vi "Set Shutter TTL.vi"(8 "error in (no error)":errorcluster, 11 "CCDCamera in":refnum<class "CCDCamera.lvclass">) -> (0 "error out":errorcluster, 3 "CCDCamera out":refnum<class "CCDCamera.lvclass">)   [LabVIEW 2018, in "CCDCamera.lvclass"]
uses:
  CCDCamera.lvclass
  C:/Users/observer/Desktop/SPARC4_ACS/SPARC4_ACS/Simulated_CCD_Camera/Simulated_CCD_Camera.lvclass
  Simulated_CCD_Camera/Simulated_CCD_Camera.lvclass/Simulated_CCD_Camera.ctl
  Interface/Interface.lvclass
  Simulated_CCD_Camera/Simulated_CCD_Camera.lvclass
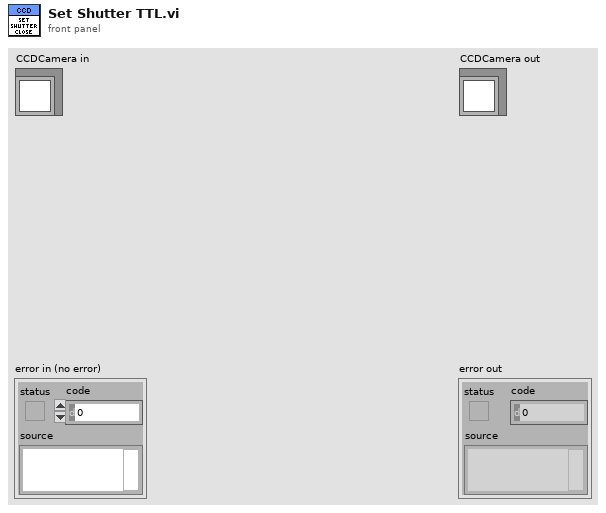
[diagram p1: front panel]
types:
  T1 = typedef "Shutter_mode typedef.ctl" = enum16{"Auto", "Open", "Close", "N/A (3)", "Open FVB Series", "Open Any Series"}
  T2 = typedef "ReadMode_mode typedef.ctl" = enum16{"Full Vertical Binning", "Multi-Track", "Random-Track", "Single-Track", "Image"}
  T3 = typedef "AcquisitionMode_mode typedef.ctl" = enum16{"Reserved (0)", "Single Scan", "Accumulate", "Kinetics", "Fast Kinetics", "Run Till Abort", "Reserved (6)", "Reserved (7)", "Reserved (8)", "Time Delayed Integration"}
  T4 = cluster{"PREAMP":enum16{"Gain 1", "Gain 2"}, "READOUT_RATE":enum16{"30 MHz", "20 MHz", "10 MHz", "1 MHz"}, "EM_GAIN":u16, "VBIN":u16, "INITIAL_LINE":u16, "INITIAL_COLUMN":u16, "FINAL_LINE":u16, "FINAL_COLUMN":u16, "TRIGGER_MODE":enum16{"Internal", "External", "N/A", "N/A_1", "N/A_2", "N/A_3", "External Start"}, "HBIN":u16, "SHUTTER_TTL":enum16{"TTL Low", "TTL High"}, "SHUTTER_MODE":T1, "SHUTTER_OPENING_TIME":u16, "SHUTTER_CLOSING_TIME":u16, "VERTICAL_SHIFT_SPEED":u16, "READ_MODE":T2, "FRAME_TRANSFER":bool, "VERTICAL_CLOCK_VOLTAGE":enum16{"0", "+1", "+2", "+3", "+4"}, "ACQUISITION_MODE":T3, "AD_CHANNEL":u16, "EM_MODE":enum16{"Electron Multiplying", "Conventional"}}
  T5 = cluster{"PREAMP":u16, "READOUT_RATE":u16, "EM_GAIN":u16, "VBIN":u16, "INITIAL_LINE":u16, "INITIAL_COLUMN":u16, "FINAL_LINE":u16, "FINAL_COLUMN":u16, "TRIGGER_MODE":u16, "HBIN":u16, "SHUTTER_TTL":u16, "SHUTTER_MODE":u16, "SHUTTER_OPENING_TIME":u16, "SHUTTER_CLOSING_TIME":u16, "VERTICAL_SHIFT_SPEED":u16, "READ_MODE":u16, "FRAME_TRANSFER":bool, "VERTICAL_CLOCK_VOLTAGE":u16, "ACQUISITION_MODE":u16, "AD_CHANNEL":u16, "EM_MODE":u16}
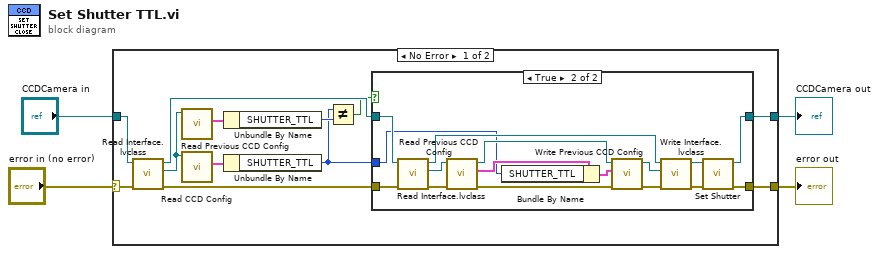
[diagram p0: block diagram]
diagram:
  n1 = case shown="No Error" "error in (no error)" {
    selector: "error in (no error)" -> [w16 w36]
    tunnel: [w13 w36] -> w1
    tunnel: [w12 w35] -> w2
    tunnel: "CCDCamera in" -> [w15 w35]
    frame No Error {
      n2 = call "Read Interface.lvclass.vi"("error in (no error)"=w16, "Simulated_CCD_Camera in"=w15) -> ("error out"=w11:errorcluster, "Interface.lvclass"=w5:refnum<class "Interface.lvclass">, "Simulated_CCD_Camera out"=w14:refnum<class "CCDCamera.lvclass">)  [unwired: 7 in]
      n3 = call "Read Previous CCD Config.vi"("Interface in"=w5) -> ("Previous CCD Config"=w9:T4)  [unwired: 8 in, 2 out]
      n4 = call "Read CCD Config.vi"("Interface in"=w5) -> ("Previous CCD Config"=w10:T5)  [unwired: 8 in, 2 out]
      n5 = Unbundle By Name(w9) -> ("SHUTTER_TTL"=w8:enum16{"TTL Low", "TTL High"})
      n6 = Unbundle By Name(w10) -> ("SHUTTER_TTL"=w6:u16)
      n7 = Not Equal?(x=w6, y=w8) -> (x != y?=w7:bool)
      n8 = case shown="True" w7 {
        tunnel: w14 -> [w18 w21]
        tunnel: [w17 w23] -> w13
        tunnel: [w18 w22] -> w12
        tunnel: w11 -> [w17 w20]
        tunnel: w6 -> [_ w19]
        frame False {
        }
        frame True {
          n9 = call "Read Interface.lvclass.vi"("error in (no error)"=w20, "Simulated_CCD_Camera in"=w21) -> ("error out"=w26:errorcluster, "Interface.lvclass"=w30:refnum<class "Interface.lvclass">, "Simulated_CCD_Camera out"=w28:refnum<class "CCDCamera.lvclass">)  [unwired: 7 in]
          n10 = call "Read Previous CCD Config.vi"("error in (no error)"=w26, "Interface in"=w30) -> ("error out"=w32:errorcluster, "Previous CCD Config"=w34:T4, "Interface out"=w31:refnum<class "Interface.lvclass">)  [unwired: 7 in]
          n11 = Bundle By Name(cluster=w34, "SHUTTER_TTL"=w19) -> (w33:T4)
          n12 = call "Write Previous CCD Config.vi"("error in (no error)"=w32, "Previous CCD Config"=w33, "Interface in"=w31) -> ("error out"=w27:errorcluster, "Interface out"=w29:refnum<class "Interface.lvclass">)  [unwired: 7 in]
          n13 = call "Write Interface.lvclass.vi"("error in (no error)"=w27, "Interface.lvclass"=w29, "Simulated_CCD_Camera in"=w28) -> ("error out"=w24:errorcluster, "Simulated_CCD_Camera out"=w25:refnum<class "CCDCamera.lvclass">)  [unwired: 7 in]
          n14 = call-dynamic "Set Shutter.vi"("error in (no error)"=w24, "CCDCamera in"=w25) -> ("error out"=w23:errorcluster, "CCDCamera out"=w22:refnum<class "CCDCamera.lvclass">)  [unwired: 8 in]
        }
      }
    }
    frame Error {
    }
  }
  "error out" <- w1
  "CCDCamera out" <- w2
